vi "Get Robot Info.vi"(8 "error in":errorcluster) -> ()   [LabVIEW 2013]
uses:
  Robot Global Data.vi
panel:
  in  "Shooter Limit Switch":bool
  in  "Simulate":bool
  in  "Current Arm Position":dbl
  in  "Lower Limit Switch":bool
  in  "Upper Limit Switch":bool
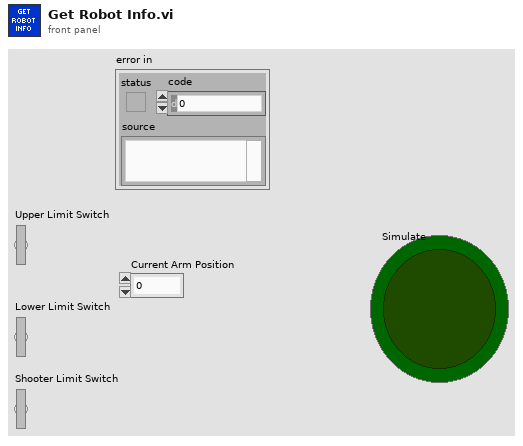
[diagram p1: front panel]
types:
  T1 = typedef "WPI_AnalogChannelDevRef.ctl" = cluster{"DevStatus":errorcluster, "Analog Module":T2, "Analog Channel":T3}
  T2 = typedef "FPGA_TypedefAnalogModule.ctl" = enum16{"Analog Module 1", "Analog Module 2"}
  T3 = typedef "FPGA_AIChannel.ctl" = enum8{"AI 1", "AI 2", "AI 3", "AI 4", "AI 5", "AI 6", "AI 7", "AI 8", "Invalid"}
  T4 = typedef "WPI_DigitalInputDevRef.ctl" = cluster{"DevStatus":errorcluster, "DIO Channel":T5, "Digital Module":T6}
  T5 = typedef "FPGA_DIOChannel.ctl" = enum8{"DIO 1", "DIO 2", "DIO 3", "DIO 4", "DIO 5", "DIO 6", "DIO 7", "DIO 8", "DIO 9", "DIO 10", "DIO 11", "DIO 12", "DIO 13", "DIO 14", "Invalid"}
  T6 = typedef "FPGA_TypedefDigitalModule.ctl" = enum16{"Digital Module 1", "Digital Module 2"}
  T7 = typedef "Robot Info Typedef.ctl" = cluster{"Arm Info":T8, "Shooter Info":T9}
  T8 = typedef "Arm Info Typedef.ctl" = cluster{"Current Arm Position":dbl, "Arm Bottom Limit Switch":bool, "Arm Top Limit Switch":bool}
  T9 = typedef "Shooter Info Typedef.ctl" = cluster{"Shooter At Full":bool}
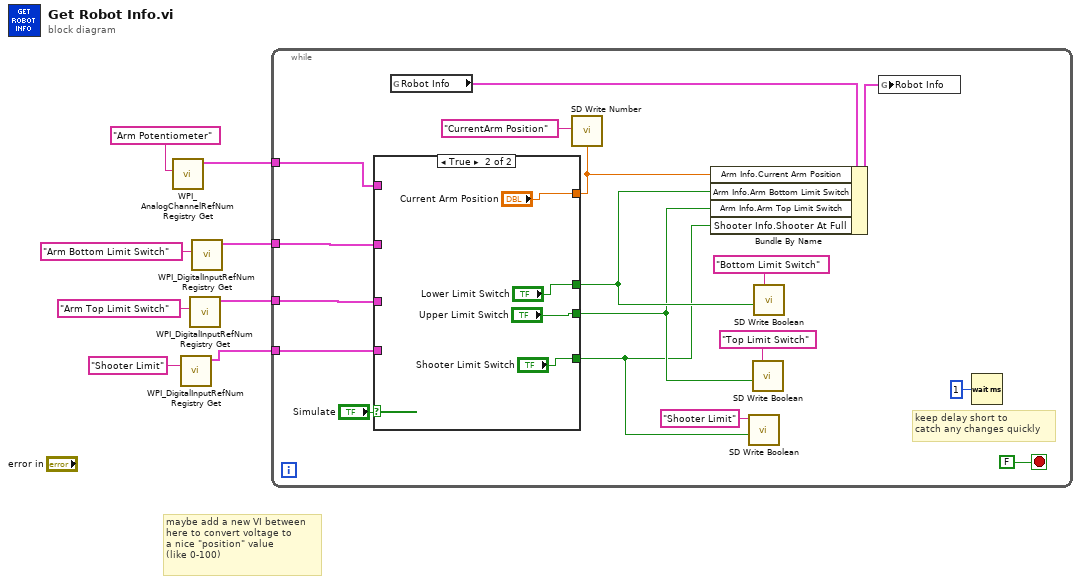
[diagram p0: block diagram]
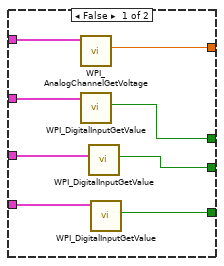
[diagram p2: hidden frame]
diagram:
  # "maybe add a new VI between\nhere to convert voltage to\na nice \"position\" value\n(like 0-100)"
  n1 = call <vilib>:"WPI_AnalogChannelRefNum Registry Get.vi"("refnum name"="Arm Potentiometer") -> ("AIDeviceRef"=w8:T1)  [unwired: 9 in, 1 out]
  n2 = call <vilib>:"WPI_DigitalInputRefNum Registry Get.vi"("refnum name"="Shooter Limit") -> ("DigitalInputDevRef"=w1:T4)  [unwired: 9 in, 1 out]
  n3 = call <vilib>:"WPI_DigitalInputRefNum Registry Get.vi"("refnum name"="Arm Top Limit Switch") -> ("DigitalInputDevRef"=w4:T4)  [unwired: 9 in, 1 out]
  n4 = call <vilib>:"WPI_DigitalInputRefNum Registry Get.vi"("refnum name"="Arm Bottom Limit Switch") -> ("DigitalInputDevRef"=w5:T4)  [unwired: 9 in, 1 out]
  n5 = while {
    tunnel: w8 -> [w22]
    tunnel: w5 -> [w18]
    tunnel: w4 -> [w17]
    tunnel: w1 -> [w11]
    stop <- FALSE stop-if-true
    # "keep delay short to\ncatch any changes quickly"
    n6 = case shown="True" "Simulate" {
      tunnel: w22 -> [w33 _]
      tunnel: [w32 "Current Arm Position"] -> w19
      tunnel: w18 -> [w31 _]
      tunnel: w17 -> [w30 _]
      tunnel: [w29 "Lower Limit Switch"] -> w16
      tunnel: [w28 "Upper Limit Switch"] -> w15
      tunnel: w11 -> [w27 _]
      tunnel: [w26 "Shooter Limit Switch"] -> w10
      frame False {
        n7 = call <vilib>:"WPI_AnalogChannelGetVoltage.vi"("AIDeviceRef"=w33) -> ("Voltage"=w32:dbl)  [unwired: 8 in, 2 out]
        n8 = call <vilib>:"WPI_DigitalInputGetValue.vi"("DigitalInputDevRef"=w31) -> ("Value"=w29:bool)  [unwired: 8 in, 2 out]
        n9 = call <vilib>:"WPI_DigitalInputGetValue.vi"("DigitalInputDevRef"=w30) -> ("Value"=w28:bool)  [unwired: 8 in, 2 out]
        n10 = call <vilib>:"WPI_DigitalInputGetValue.vi"("DigitalInputDevRef"=w27) -> ("Value"=w26:bool)  [unwired: 8 in, 2 out]
      }
      frame True {
      }
    }
    n11 = global read "Robot Global Data.vi" "Robot Info"() -> (w24:T7)
    n12 = call <vilib>:"SD Write Number.vi"("Numeric"=w19, "Name"="CurrentArm Position") -> ()  [unwired: 8 in, 2 out]
    n13 = Bundle By Name(cluster=w24, "Arm Info.Current Arm Position"=w19, "Arm Info.Arm Bottom Limit Switch"=w16, "Arm Info.Arm Top Limit Switch"=w15, "Shooter Info.Shooter At Full"=w10) -> (w23:T7)
    n14 = call <vilib>:"SD Write Boolean.vi"("Boolean"=w10, "Name"="Shooter Limit") -> ()  [unwired: 8 in, 2 out]
    n15 = call <vilib>:"SD Write Boolean.vi"("Boolean"=w15, "Name"="Top Limit Switch") -> ()  [unwired: 8 in, 2 out]
    n16 = call <vilib>:"SD Write Boolean.vi"("Boolean"=w16, "Name"="Bottom Limit Switch") -> ()  [unwired: 8 in, 2 out]
    n17 = global write "Robot Global Data.vi" "Robot Info"(w23) -> ()
    n18 = Wait (ms)(milliseconds to wait=u32 1) -> ()  [unwired: 1 out]
  }
